vi "svx_Scale Num Plots.vi"(7 "Display State In":T1={"X Scale Width %"=50.0, "Y Scale Height %"=50.0, "X-Axis Range"={"Minimum"=0.0, "Maximum"=10.0}, "Y-Axis Range"={"Minimum"=0.0, "Maximum"=10.0}, "Z-Axis Range"={"Minimum"=0.0, "Maximum"=10.0}, "Plot Color"=61212, "Frame Color"=16252785, "Background Color"=16777222, "Initial AutoScale Y"=TRUE, "AutoScale X"=2, "AutoScale Y"=2, "AutoScale Z"=2, "Plot Transparency"=FALSE, "X-Axis Name"="Frequency", "Y-Axis Name"="Amplitude", "Z-Axis Name"="", "X-Axis Scaling Factor"={"Offset"=0.0, "Multiplier"=1.0}, "Y-Axis Scaling Factor"={"Offset"=0.0, "Multiplier"=1.0}, "Z-Axis Scaling Factor"={"Offset"=0.0, "Multiplier"=1.0}, "X-Scale Visible"=TRUE, "Y-Scale Visible"=TRUE, "Z-Scale Visible"=TRUE, "X-Scale Label Visible"=TRUE, "Y-Scale Label Visible"=TRUE, "Z-Scale Label Visible"=TRUE, "X-Axis Range Scaled"={"Minimum"=0.0, "Maximum"=10.0}, "Y-Axis Range Scaled"={"Minimum"=0.0, "Maximum"=10.0}, "Z-Axis Range Scaled"={"Minimum"=0.0, "Maximum"=10.0}, "Rev Z Order"=FALSE, "X-Scale Format Str"="%#.4g", "Y-Scale Format Str"="%#.4g", "Z-Scale Format Str"="%#.4g", "Decor color"=12369084, "Scale Range Change"=refnum, "out of state queue"=refnum, "property nodes"=refnum, "Lines"=[], "Line Properties"={"Line Color"=61212, "Line Width"=61212, "Line Style"=enum."Dash", "DisplayLines"=FALSE}} caption="State" {"Line Properties"."Line Width" min=1}, 9 "dz":dbl=1.0, 10 "z0":dbl, 11 "Plots":cluster{"x0":dbl, "dx":dbl, "Y":dbl[]}[](array[cluster])) -> (1 "Z length":i32, 2 "Z Index":i32, 3 "Plots out":cluster{"x0":dbl, "dx":dbl, "Y":dbl[]}[](array[cluster]))   [LabVIEW 2017, in "SVX Waterfall Graph.xctl"]
uses:
  <vilib>/addons/_XControls/Waterfall Graph/SVX Waterfall Graph.xctl
  <vilib>/addons/_XControls/Waterfall Graph/subVIs/svx_Waterfall State.ctl
  <vilib>/addons/_NISVFA/_Shared subVIs/Controls/svc_Cluster of Array of Cluster of XYZ.ctl
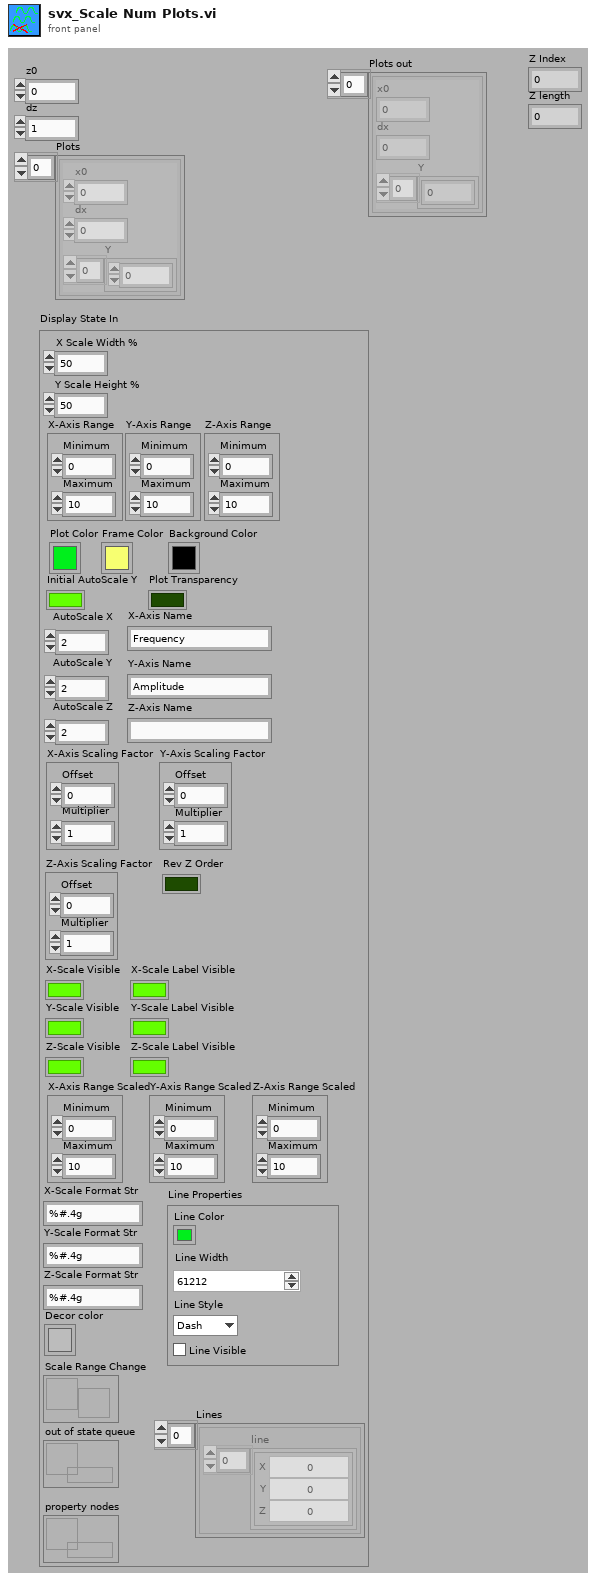
[diagram p1: front panel]
types:
  T1 = typedef "SVX Waterfall Graph.xctl/svx_Waterfall State.ctl" = cluster{"X Scale Width %":dbl, "Y Scale Height %":dbl, "X-Axis Range":cluster{"Minimum":dbl, "Maximum":dbl}, "Y-Axis Range":cluster{"Minimum":dbl, "Maximum":dbl}, "Z-Axis Range":cluster{"Minimum":dbl, "Maximum":dbl}, "Plot Color":u32, "Frame Color":u32, "Background Color":u32, "Initial AutoScale Y":bool, "AutoScale X":u8, "AutoScale Y":u8, "AutoScale Z":u8, "Plot Transparency":bool, "X-Axis Name":string, "Y-Axis Name":string, "Z-Axis Name":string, "X-Axis Scaling Factor":cluster{"Offset":dbl, "Multiplier":dbl}, "Y-Axis Scaling Factor":cluster{"Offset":dbl, "Multiplier":dbl}, "Z-Axis Scaling Factor":cluster{"Offset":dbl, "Multiplier":dbl}, "X-Scale Visible":bool, "Y-Scale Visible":bool, "Z-Scale Visible":bool, "X-Scale Label Visible":bool, "Y-Scale Label Visible":bool, "Z-Scale Label Visible":bool, "X-Axis Range Scaled":cluster{"Minimum":dbl, "Maximum":dbl}, "Y-Axis Range Scaled":cluster{"Minimum":dbl, "Maximum":dbl}, "Z-Axis Range Scaled":cluster{"Minimum":dbl, "Maximum":dbl}, "Rev Z Order":bool, "X-Scale Format Str":string, "Y-Scale Format Str":string, "Z-Scale Format Str":string, "Decor color":u32, "Scale Range Change":refnum<user-event>, "out of state queue":refnum<queue>, "property nodes":refnum<queue>, "Lines":T2[], "Line Properties":cluster{"Line Color":u32, "Line Width":u16, "Line Style":enum32{"Solid", "Dash", "Dot", "DashDot", "DashDotDot"}, "DisplayLines":bool}}
  T2 = typedef "svc_Cluster of Array of Cluster of XYZ.ctl" = cluster{"line":cluster{"X":dbl, "Y":dbl, "Z":dbl}[]}
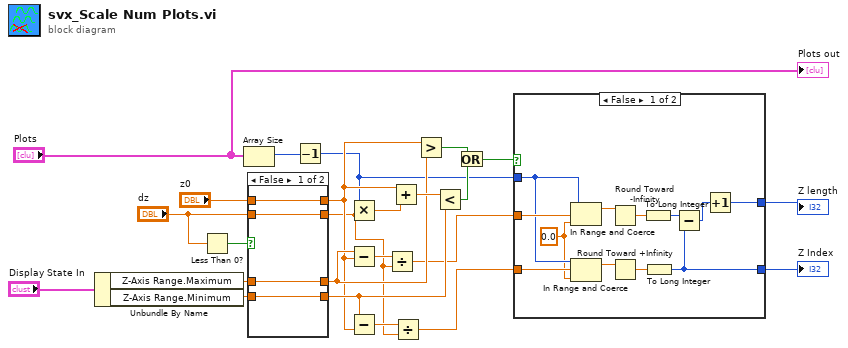
[diagram p0: block diagram]
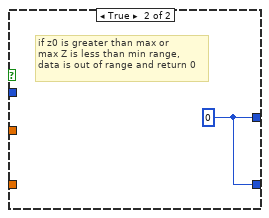
[diagram p2: hidden frame]
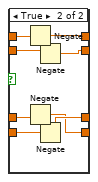
[diagram p3: hidden frame]
diagram:
  n1 = Unbundle By Name("Display State In") -> ("Z-Axis Range.Maximum"=w20:dbl, "Z-Axis Range.Minimum"=w19:dbl)
  n2 = Less Than 0?(x="dz") -> (x < 0?=w21:bool)
  n3 = Array Size(array="Plots") -> (size(s)=w13:i32)
  n4 = case shown="False" w21 {
    tunnel: "z0" -> [w28 w36]
    tunnel: [w28 w35] -> w8
    tunnel: "dz" -> [w27 w34]
    tunnel: [w27 w33] -> w6
    tunnel: w20 -> [w26 w32]
    tunnel: w19 -> [w25 w31]
    tunnel: [w26 w30] -> w12
    tunnel: [w25 w29] -> w9
    frame False {
    }
    frame True {
      n5 = Negate(x=w36) -> (-x=w35:dbl)
      n6 = Negate(x=w32) -> (-x=w29:dbl)
      n7 = Negate(x=w34) -> (-x=w33:dbl)
      n8 = Negate(x=w31) -> (-x=w30:dbl)
    }
  }
  n9 = Decrement(x=w13) -> (x-1=w4:i32)
  n10 = Multiply(x=w4, y=w6) -> (x*y=w14:dbl)
  n11 = Subtract(x=w12, y=w8) -> (x-y=w11:dbl)
  n12 = Subtract(x=w9, y=w8) -> (x-y=w10:dbl)
  n13 = Divide(x=w11, y=w6) -> (x/y=w5:dbl)
  n14 = Add(x=w8, y=w14) -> (x+y=w18:dbl)
  n15 = Divide(x=w10, y=w6) -> (x/y=w7:dbl)
  n16 = Greater?(x=w8, y=w12) -> (0:w17:bool)
  n17 = Less?(x=w18, y=w9) -> (x < y?=w16:bool)
  n18 = Or(x=w17, y=w16) -> (x .or. y?=w15:bool)
  n19 = case shown="False" w15 {
    tunnel: w5 -> [w45 _]
    tunnel: w7 -> [w44 _]
    tunnel: w4 -> [w42 _]
    tunnel: [w40 w49] -> w22
    tunnel: [w37 w49] -> w23
    frame False {
      w41 = 0.0 ("lower limit")
      n20 = In Range and Coerce(upper limit=w42, x=w45, lower limit=w41) -> (coerced(x)=w46:dbl)  [unwired: 1 out]
      n21 = In Range and Coerce(upper limit=w42, x=w44, lower limit=w41) -> (coerced(x)=w43:dbl)  [unwired: 1 out]
      n22 = Round Toward -Infinity(1:w46) -> (0:w48:dbl)
      n23 = Round Toward +Infinity(x=w43) -> (ceil(x): smallest int >= x=w39:dbl)
      n24 = To Long Integer(number=w48) -> (32bit integer=w38:i32)
      n25 = To Long Integer(number=w39) -> (32bit integer=w37:i32)
      n26 = Subtract(x=w38, y=w37) -> (x-y=w47:i32)
      n27 = Increment(x=w47) -> (x+1=w40:i32)
    }
    frame True {
      w49 = 0
      # "if z0 is greater than max or\nmax Z is less than min range,\ndata is out of range and return 0"
    }
  }
  "Z Index" <- w23
  "Z length" <- w22
  "Plots out" <- "Plots"
